vi "flatten and unflatten test.vi"() -> ()   [LabVIEW 2014, in "Tagbus PID Module tests.lvlib"]
uses:
  testing/Tagbus PID Module tests.lvlib
  PID Loop.lvclass
panel:
  out "output range":cluster{"output high":dbl, "output low":dbl}
  out "PID gains":T1
  out "PID Parameters":T2
  out "ID":string
  out "error out":errorcluster
  in  "error in (no error)":errorcluster
  out "flattened PID Loop":string
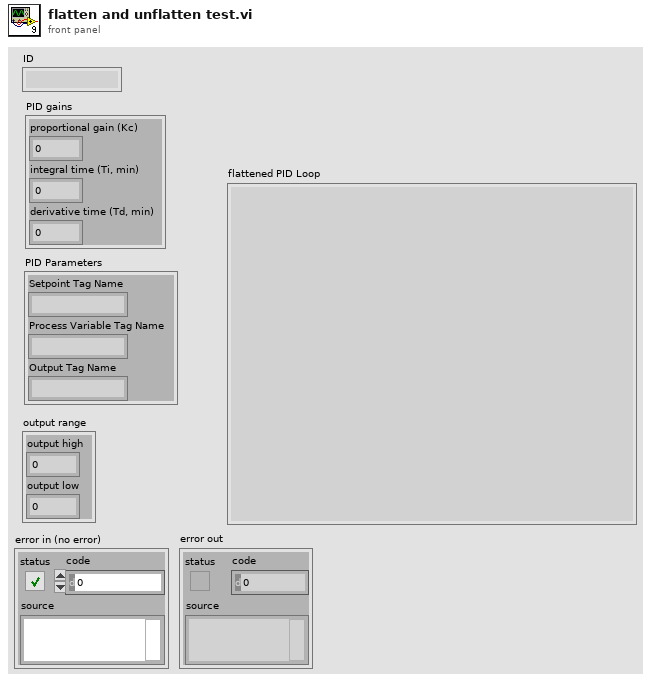
[diagram p1: front panel]
types:
  T1 = cluster{"proportional gain (Kc)":dbl, "integral time (Ti, min)":dbl, "derivative time (Td, min)":dbl}
  T2 = cluster{"Setpoint Tag Name":string, "Process Variable Tag Name":string, "Output Tag Name":string}
  T3 = typedef "PID Parameters.ctl" = cluster{"Setpoint Tag":string, "Process Variable Tag":string, "Output Tag":string}
  T4 = typedef "PID Gains.ctl" = cluster{"proportional gain (Kc)":dbl, "integral time (Ti, min)":dbl, "derivative time (Td, min)":dbl}
  T5 = typedef "PID Range.ctl" = cluster{"output high":dbl, "output low":dbl}
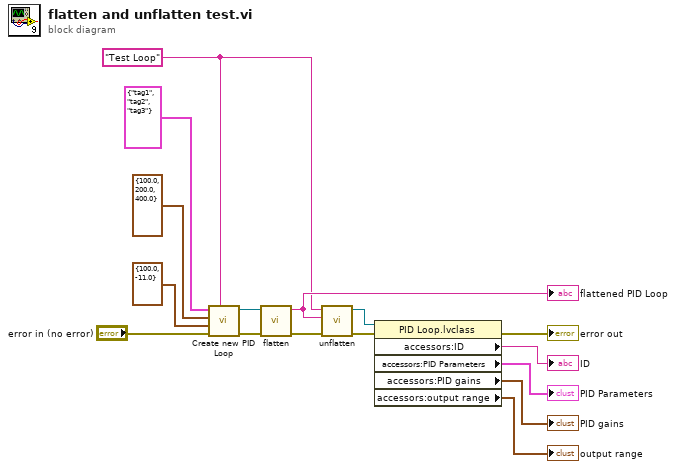
[diagram p0: block diagram]
diagram:
  w8 = "Test Loop" ("ID")
  n1 = call "Create new PID Loop.vi"("ID"=w8, "error in (no error)"="error in (no error)", "output range"=cluster{"output high":dbl, "output low":dbl} {"output high"=100.0, "output low"=-11.0}, "PID gains"=T1 {"proportional gain (Kc)"=100.0, "integral time (Ti, min)"=200.0, "derivative time (Td, min)"=400.0}, "PID Parameters"=T2 {"Setpoint Tag Name"="tag1", "Process Variable Tag Name"="tag2", "Output Tag Name"="tag3"}) -> ("error out"=w15:errorcluster, "PID Loop out"=w16:refnum<class "PID Loop.lvclass">)  [unwired: 5 in]
  n2 = call-dynamic "flatten.vi"("error in (no error)"=w15, "PID Loop in"=w16) -> ("error out"=w10:errorcluster, "flattened PID Loop"=w9:string)  [unwired: 8 in]
  "flattened PID Loop" <- w9
  n3 = call "unflatten.vi"("error in (no error)"=w10, "PID Loop String"=w9, "Identifier"=w8) -> ("error out"=w5:errorcluster, "PID Loop out"=w7:refnum<class "PID Loop.lvclass">)  [unwired: 7 in]
  n4 = property class="PID Loop.lvclass"(reference=w7, error in=w5) -> (error out=→"error out":errorcluster, "accessors:ID"=→"ID":string, "accessors:PID Parameters"=→"PID Parameters":T3, "accessors:PID gains"=→"PID gains":T4, "accessors:output range"=→"output range":T5)  [unwired: 1 out]
